vi "Pasco Excel Write.vi"(5 "Folder Location":string, 7 "File Name":string, 8 "WriteToExcel":bool, 9 "Save Data":bool, 10 "PIDARRAY":dbl[][](array[numeric]), 11 "EncoderRate":dbl) -> (3 "Sent?":string="File Wrote")   [LabVIEW 2011]
uses:
  <vilib>/Utility/file.llb/Write To Spreadsheet File (DBL).vi
panel:
  out "new file path (Not A Path if cancelled)":path
  out "path":path
  out "RateMeasurement":dbl
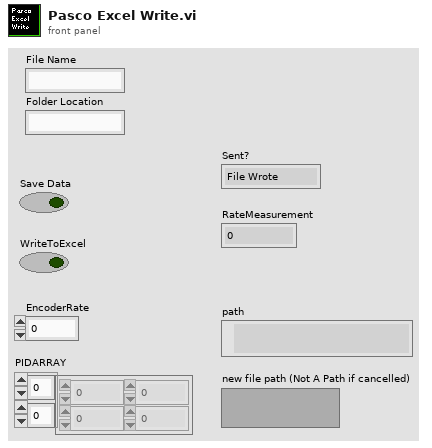
[diagram p1: front panel]
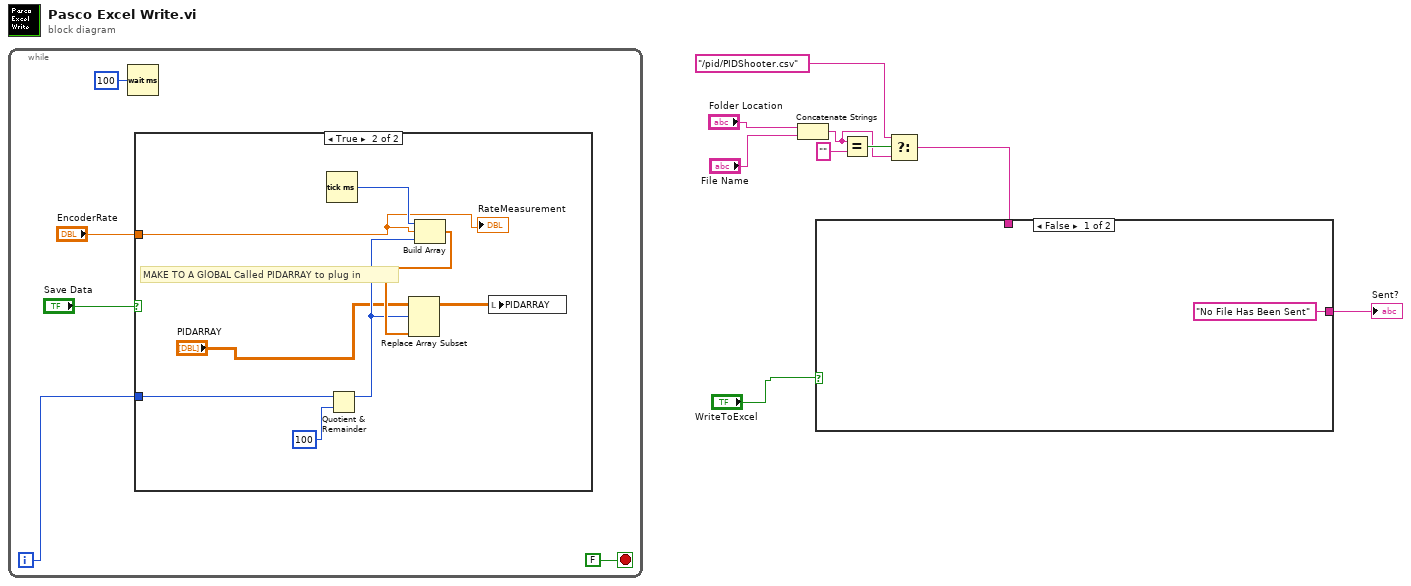
[diagram p0: block diagram]
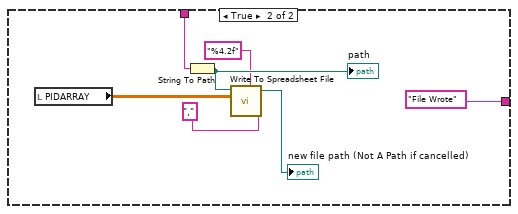
[diagram p2: hidden frame]
diagram:
  n1 = while {
    i -> [w13]
    stop <- FALSE stop-if-true
    n2 = Wait (ms)(milliseconds to wait=u32 100) -> ()  [unwired: 1 out]
    n3 = case shown="True" "Save Data" {
      tunnel: w13 -> [_ w18]
      tunnel: "EncoderRate" -> [_ w17]
      frame False {
      }
      frame True {
        # "MAKE TO A GlOBAL Called PIDARRAY to plug in"
        n4 = Tick Count (ms)() -> (millisecond timer value=w21:u32)
        n5 = Quotient & Remainder(x=w18, y=100) -> (x-y*floor(x/y)=w19:i32)  [unwired: 1 out]
        n6 = Build Array(w21, w17, w19) -> (w22:dbl[])
        n7 = Replace Array Subset(array="PIDARRAY", new element=w22, index (row)=w19) -> (w15:dbl[][])  [unwired: 1 in]
        n8 = local write "PIDARRAY"(w15) -> ()
        "RateMeasurement" <- w17
      }
    }
  }
  n9 = Concatenate Strings("Folder Location", "File Name") -> (w2:string)
  n10 = Equal?(x=w2, y="") -> (x = y?=w4:bool)
  n11 = Select(t="/pid/PIDShooter.csv" ("string"), s=w4, f=w2) -> (s? t:f=w1:string)
  n12 = case shown="False" "WriteToExcel" {
    tunnel: ["No File Has Been Sent" "File Wrote"] -> w8
    tunnel: w1 -> [_ w24]
    frame False {
    }
    frame True {
      n13 = local read "PIDARRAY"() -> (w26:dbl[][])
      n14 = String To Path(string=w24) -> (path=w30:path)
      "path" <- w30
      n15 = call-poly <vilib>:"Write To Spreadsheet File.vi"("delimiter (\\t)"="," ("delimiter (\\t)"), "format (%.3f)"="%4.2f", "2D data"=w26, "file path (dialog if empty)"=w30) -> ("new file path (Not A Path if cancelled)"=→"new file path (Not A Path if cancelled)":path)  [unwired: 4 in]
    }
  }
  "Sent?" <- w8
